vi "F2Machine.vi"   [LabVIEW 2011]
uses:
  API/API DYM.lvlib
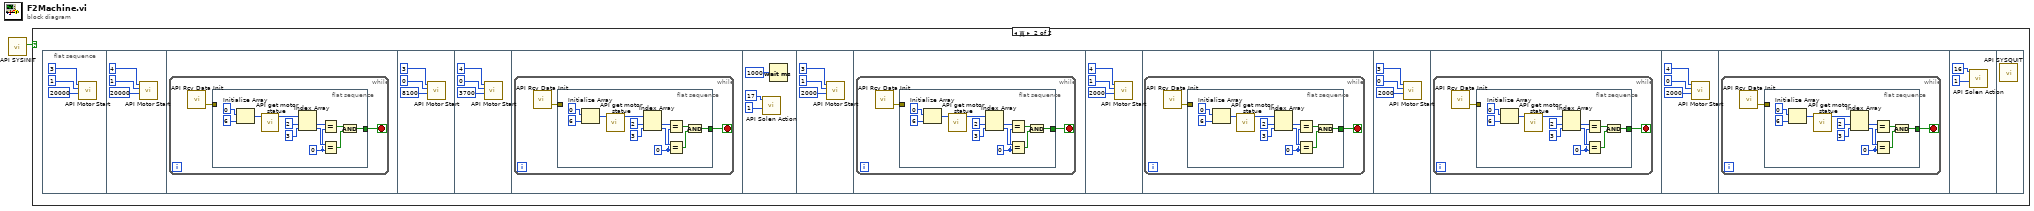
[diagram p0: block diagram]
diagram:
  n1 = call "API SYSINIT.vi"() -> ("SYSINIT return value"=w1:bool)  [unwired: 11 in]
  n2 = case shown="真" w1 {
    frame False {
    }
    frame True {
      n3 = flat-sequence {
        frame #0 {
          n4 = call "API Motor Start.vi"("stepNum"=20000, "direction"=1, "motorNum"=3) -> ()  [unwired: 8 in, 1 out]
        }
        frame #1 {
          n5 = call "API Motor Start.vi"("stepNum"=20000, "direction"=1, "motorNum"=4) -> ()  [unwired: 8 in, 1 out]
        }
        frame #2 {
          n6 = while {
            stop <- w8 stop-if-true
            n7 = call "API Rcv Data Init.vi"() -> ("错误输出"=w9:errorcluster)  [unwired: 2 in, 1 out]
            n8 = flat-sequence {
              tunnel: w9 -> [_]
              tunnel: [w10] -> w8
              frame #0 {
                w13 = 0
                n9 = Initialize Array(0 ("元素"), 6 ("维数大小")) -> (w19:i32[])
                n10 = call "API get motor statue.vi"("motor statue array input"=w19) -> ("motor statue array output"=w18:i32[])  [unwired: 9 in, 1 out]
                n11 = Index Array(array=w18, index #1=2 ("索引"), index #2=3 ("索引")) -> (element #1=w15:i32, element #2=w14:i32)
                n12 = Equal?(x=w15, y=w13) -> (x = y?=w12:bool)
                n13 = Equal?(x=w14, y=w13) -> (x = y?=w11:bool)
                n14 = And(x=w12, y=w11) -> (x .and. y?=w10:bool)
              }
            }
          }
        }
        frame #3 {
          n15 = call "API Motor Start.vi"("stepNum"=8100, "direction"=0, "motorNum"=3) -> ()  [unwired: 8 in, 1 out]
        }
        frame #4 {
          n16 = call "API Motor Start.vi"("stepNum"=3700, "direction"=0, "motorNum"=4) -> ()  [unwired: 8 in, 1 out]
        }
        frame #5 {
          n17 = while {
            stop <- w28 stop-if-true
            n18 = call "API Rcv Data Init.vi"() -> ("错误输出"=w29:errorcluster)  [unwired: 2 in, 1 out]
            n19 = flat-sequence {
              tunnel: w29 -> [_]
              tunnel: [w30] -> w28
              frame #0 {
                w33 = 0
                n20 = Initialize Array(0 ("元素"), 6 ("维数大小")) -> (w39:i32[])
                n21 = call "API get motor statue.vi"("motor statue array input"=w39) -> ("motor statue array output"=w38:i32[])  [unwired: 9 in, 1 out]
                n22 = Index Array(array=w38, index #1=2 ("索引"), index #2=3 ("索引")) -> (element #1=w35:i32, element #2=w34:i32)
                n23 = Equal?(x=w35, y=w33) -> (x = y?=w32:bool)
                n24 = Equal?(x=w34, y=w33) -> (x = y?=w31:bool)
                n25 = And(x=w32, y=w31) -> (x .and. y?=w30:bool)
              }
            }
          }
        }
        frame #6 {
          n26 = call "API Solen Action.vi"("statue"=1, "solenNum"=17) -> ()  [unwired: 9 in, 1 out]
          n27 = Wait (ms)(milliseconds to wait=u32 1000 ("等待时间（毫秒）")) -> ()  [unwired: 1 out]
        }
        frame #7 {
          n28 = call "API Motor Start.vi"("stepNum"=2000, "direction"=1, "motorNum"=3) -> ()  [unwired: 8 in, 1 out]
        }
        frame #8 {
          n29 = while {
            stop <- w48 stop-if-true
            n30 = call "API Rcv Data Init.vi"() -> ("错误输出"=w49:errorcluster)  [unwired: 2 in, 1 out]
            n31 = flat-sequence {
              tunnel: w49 -> [_]
              tunnel: [w50] -> w48
              frame #0 {
                w53 = 0
                n32 = Initialize Array(0 ("元素"), 6 ("维数大小")) -> (w59:i32[])
                n33 = call "API get motor statue.vi"("motor statue array input"=w59) -> ("motor statue array output"=w58:i32[])  [unwired: 9 in, 1 out]
                n34 = Index Array(array=w58, index #1=2 ("索引"), index #2=3 ("索引")) -> (element #1=w55:i32, element #2=w54:i32)
                n35 = Equal?(x=w55, y=w53) -> (x = y?=w52:bool)
                n36 = Equal?(x=w54, y=w53) -> (x = y?=w51:bool)
                n37 = And(x=w52, y=w51) -> (x .and. y?=w50:bool)
              }
            }
          }
        }
        frame #9 {
          n38 = call "API Motor Start.vi"("stepNum"=2000, "direction"=1, "motorNum"=4) -> ()  [unwired: 8 in, 1 out]
        }
        frame #10 {
          n39 = while {
            stop <- w65 stop-if-true
            n40 = call "API Rcv Data Init.vi"() -> ("错误输出"=w66:errorcluster)  [unwired: 2 in, 1 out]
            n41 = flat-sequence {
              tunnel: w66 -> [_]
              tunnel: [w67] -> w65
              frame #0 {
                w70 = 0
                n42 = Initialize Array(0 ("元素"), 6 ("维数大小")) -> (w76:i32[])
                n43 = call "API get motor statue.vi"("motor statue array input"=w76) -> ("motor statue array output"=w75:i32[])  [unwired: 9 in, 1 out]
                n44 = Index Array(array=w75, index #1=2 ("索引"), index #2=3 ("索引")) -> (element #1=w72:i32, element #2=w71:i32)
                n45 = Equal?(x=w72, y=w70) -> (x = y?=w69:bool)
                n46 = Equal?(x=w71, y=w70) -> (x = y?=w68:bool)
                n47 = And(x=w69, y=w68) -> (x .and. y?=w67:bool)
              }
            }
          }
        }
        frame #11 {
          n48 = call "API Motor Start.vi"("stepNum"=2000, "direction"=0, "motorNum"=3) -> ()  [unwired: 8 in, 1 out]
        }
        frame #12 {
          n49 = while {
            stop <- w82 stop-if-true
            n50 = call "API Rcv Data Init.vi"() -> ("错误输出"=w83:errorcluster)  [unwired: 2 in, 1 out]
            n51 = flat-sequence {
              tunnel: w83 -> [_]
              tunnel: [w84] -> w82
              frame #0 {
                w87 = 0
                n52 = Initialize Array(0 ("元素"), 6 ("维数大小")) -> (w93:i32[])
                n53 = call "API get motor statue.vi"("motor statue array input"=w93) -> ("motor statue array output"=w92:i32[])  [unwired: 9 in, 1 out]
                n54 = Index Array(array=w92, index #1=2 ("索引"), index #2=3 ("索引")) -> (element #1=w89:i32, element #2=w88:i32)
                n55 = Equal?(x=w89, y=w87) -> (x = y?=w86:bool)
                n56 = Equal?(x=w88, y=w87) -> (x = y?=w85:bool)
                n57 = And(x=w86, y=w85) -> (x .and. y?=w84:bool)
              }
            }
          }
        }
        frame #13 {
          n58 = call "API Motor Start.vi"("stepNum"=2000, "direction"=0, "motorNum"=4) -> ()  [unwired: 8 in, 1 out]
        }
        frame #14 {
          n59 = while {
            stop <- w99 stop-if-true
            n60 = call "API Rcv Data Init.vi"() -> ("错误输出"=w100:errorcluster)  [unwired: 2 in, 1 out]
            n61 = flat-sequence {
              tunnel: w100 -> [_]
              tunnel: [w101] -> w99
              frame #0 {
                w104 = 0
                n62 = Initialize Array(0 ("元素"), 6 ("维数大小")) -> (w110:i32[])
                n63 = call "API get motor statue.vi"("motor statue array input"=w110) -> ("motor statue array output"=w109:i32[])  [unwired: 9 in, 1 out]
                n64 = Index Array(array=w109, index #1=2 ("索引"), index #2=3 ("索引")) -> (element #1=w106:i32, element #2=w105:i32)
                n65 = Equal?(x=w106, y=w104) -> (x = y?=w103:bool)
                n66 = Equal?(x=w105, y=w104) -> (x = y?=w102:bool)
                n67 = And(x=w103, y=w102) -> (x .and. y?=w101:bool)
              }
            }
          }
        }
        frame #15 {
          n68 = call "API Solen Action.vi"("statue"=1, "solenNum"=16) -> ()  [unwired: 9 in, 1 out]
        }
        frame #16 {
          n69 = call "API SYSQUIT.vi"() -> ()  [unwired: 12 in]
        }
      }
    }
  }
